vi "StopRequest.vi"(8 "error in (no error)":errorcluster, 9 "Wait for Module to stop? (F)":bool, 11 "ModuleAdminIn":refnum<class "ModuleAdmin.lvclass">) -> (0 "error out":errorcluster, 2 "Wait to Stop":bool, 3 "ModuleAdminOut":refnum<class "ModuleAdmin.lvclass">)   [LabVIEW 2018, in "AcPwrModule.lvlib"]
doc: "This VI sends an event to to any event structure listening to indicate that the module controlling the instrument should stop the module from running and close the module. If the module is currently controlling the instrument then before the module is stoped and closed the instruments acquisiton/genration/measurment acquisiton is stopped, and the conneciton to the instrument is closed."
uses:
  AcPwrModule.lvlib
  <userlib>/NIST/ModuleAdminLib/ModuleAdmin/ModuleAdmin.lvclass
  <vilib>/event_ctls.llb/usereventprio.ctl
  AcPwrShared/clStopArgument.ctl
  AcPwrShared/clEventType.ctl
  AcPwrShared/AcPwrShared.lvlib
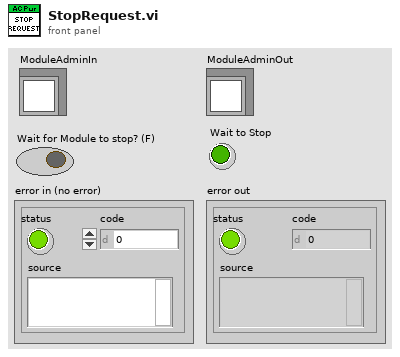
[diagram p1: front panel]
types:
  T1 = typedef "AcPwrShared.lvlib/clRequestEvents.ctl" = cluster{"StopRequest":refnum<user-event>, "PathToINI":refnum<user-event>, " LoadPlugin":refnum<user-event>, "ShowPanel":refnum<user-event>, "PrefDlg":refnum<user-event>, "InitAcPwr":refnum<user-event>, "Reset":refnum<user-event>, "Close":refnum<user-event>, "StopMeas":refnum<user-event>, "StartMeas":refnum<user-event>, "ConfigDevice":refnum<user-event>, "DeviceOn":refnum<user-event>, "DeviceOff":refnum<user-event>, "GetSettings":refnum<user-event>, "SetSettings":refnum<user-event>}
  T2 = typedef "AcPwrShared.lvlib/clEventType.ctl" = cluster{"ModuleID":i32, "Data":variant}
  T3 = typedef "AcPwrShared.lvlib/clStopArgument.ctl" = cluster{"Exit via Stop Module Req?":bool, "Wait for Module to stop?":bool, "ModuleAdmin":refnum<class "ModuleAdmin.lvclass">}
  T4 = typedef "usereventprio.ctl" = enum32{"high priority", "normal priority"}
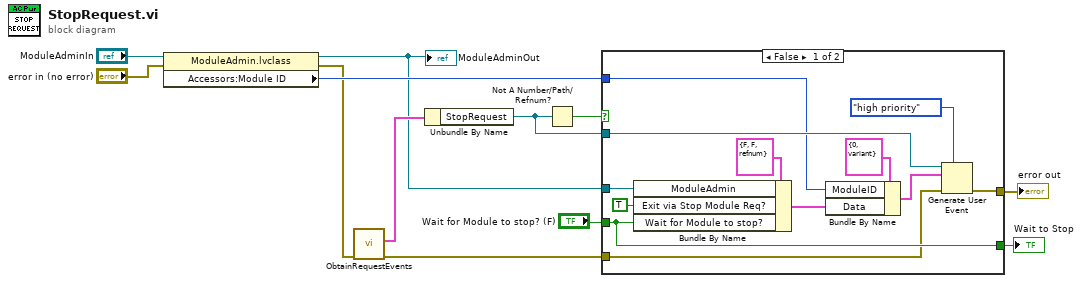
[diagram p0: block diagram]
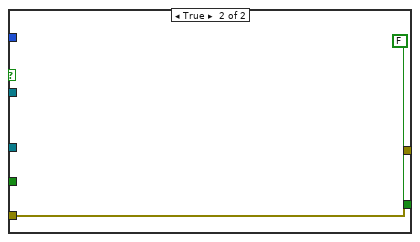
[diagram p2: hidden frame]
diagram:
  n1 = property class="ModuleAdmin.lvclass"(reference="ModuleAdminIn", error in="error in (no error)") -> (reference out=w1:refnum<class "ModuleAdmin.lvclass">, error out=w4:errorcluster, "Accessors:Module ID"=w7:i32)
  "ModuleAdminOut" <- w1
  n2 = call "ObtainRequestEvents.vi"("error in (no error)"=w4) -> ("error out"=w2:errorcluster, "clRequestEvents"=w12:T1)  [unwired: 9 in]
  n3 = Unbundle By Name(w12) -> ("StopRequest"=w10:refnum<user-event>)
  n4 = Not A Number/Path/Refnum?(number/path/refnum=w10) -> (NaN/Path/Refnum?=w11:bool)
  n5 = case shown="False" w11 {
    tunnel: w10 -> [w24 _]
    tunnel: w1 -> [w17 _]
    tunnel: "Wait for Module to stop? (F)" -> [w14 _]
    tunnel: [w16 w25] -> w5
    tunnel: w7 -> [w15 _]
    tunnel: [w14 FALSE] -> w6
    tunnel: w2 -> [w13 w25]
    frame False {
      n6 = Bundle By Name(cluster=T3 {"Exit via Stop Module Req?"=FALSE, "Wait for Module to stop?"=FALSE, "ModuleAdmin"=refnum} ("Stop Argument"), "ModuleAdmin"=w17, "Exit via Stop Module Req?"=TRUE, "Wait for Module to stop?"=w14) -> (w19:T3)
      n7 = Bundle By Name(cluster=T2 {"ModuleID"=0, "Data"=variant} ("clBroadcast"), "ModuleID"=w15, "Data"=w19) -> (w18:T2)
      n8 = Generate User Event(priority (normal)=usereventprio."high priority", user event=w24, event data cluster=w18, error in=w13) -> (error out=w16:errorcluster)  [unwired: 1 out]
    }
    frame True {
    }
  }
  "error out" <- w5
  "Wait to Stop" <- w6
